vi "SwerveDrivePoseEst_UpdateWithTime.vi"(6 "ModulePositions":T1[](array[typedef]) {"Angle"."SIN" format="%13.4f"; "Angle"."COS" format="%13.4f"; "Angle"."VALUE" format="%13.4f"}, 8 "SweveModuleStates":T3[](array[typedef]) {"Angle"."SIN" format="%13.4f"; "Angle"."COS" format="%13.4f"; "Angle"."VALUE" format="%13.4f"}, 9 "GyroAngle":T2={"VALUE"=0.0, "COS"=1.0, "SIN"=0.0} {"SIN" format="%13.4f"; "COS" format="%13.4f"; "VALUE" format="%13.4f"}, 10 "CurrentTimeSeconds":dbl, 11 "in SwerveDrivePoseEstimate":T6={"M_VisionContR"=[], "m_nominal_dT"=0.0, "m_PrevTime_Sec"=0.0, "m_GyroOffset"={"VALUE"=0.0, "COS"=1.0, "SIN"=0.0}, "m_PrevAngle"={"VALUE"=0.0, "COS"=1.0, "SIN"=0.0}, "m_Observer"={"m_P"=[], "m_xHat"=[], "States"=0, "Outputs"=0, "m_ContR"=[], "m_ContQ"=[], "m_SigmasF"=[], "m_dT_Sec"=0.0, "MERWE_SCALED_SIGMA_PTS"={"m_Wm"=[], "States"=0, "Alpha"=0.0, "m_Wc"=[], "Kappa"=0}, "meanFuncX"=refnum, "meanFuncY"=refnum, "residualFuncX"=refnum, "residualFuncY"=refnum, "addFuncX"=refnum, "addFuncXExtra"=variant, "residualFuncYExtra"=variant, "residualFuncXExtra"=variant, "MeanFuncYExtra"=variant, "MeanFuncXExtra"=variant, "Inputs"=0}, "m_kinematics"={"NumModules"=0, "InverseKinematics"=[], "ForwardKinematics"=[], "Modules"=[], "PrevCoR"={"X"=0.0, "Y"=0.0}, "SavedModuleStates"=[]}, "Pose_Buffer"={"TimeStamps"=[], "Pose"=[], "Min_TimeStamp"=0.0, "Max_TimeStamp"=0.0, "ItemCount"=0, "MaxBufferTime"=0.0}, "States"=0, "Inputs"=0, "Outputs"=0} {"Pose_Buffer"."Pose"."ROTATION"."SIN" format="%13.4f"; "Pose_Buffer"."Pose"."ROTATION"."COS" format="%13.4f"; "Pose_Buffer"."Pose"."ROTATION"."VALUE" format="%13.4f"; "Pose_Buffer"."Pose"."TRANSLATION"."Y" format="%14.3f"; "Pose_Buffer"."Pose"."TRANSLATION"."X" format="%14.3f"; "m_kinematics"."SavedModuleStates"."Angle"."SIN" format="%13.4f"; "m_kinematics"."SavedModuleStates"."Angle"."COS" format="%13.4f"; "m_kinematics"."SavedModuleStates"."Angle"."VALUE" format="%13.4f"; "m_kinematics"."PrevCoR"."Y" format="%14.3f"; "m_kinematics"."PrevCoR"."X" format="%14.3f"; "m_kinematics"."Modules"."Y" format="%14.3f"; "m_kinematics"."Modules"."X" format="%14.3f"; "m_PrevAngle"."SIN" format="%13.4f"; "m_PrevAngle"."COS" format="%13.4f"; "m_PrevAngle"."VALUE" format="%13.4f"; "m_GyroOffset"."SIN" format="%13.4f"; "m_GyroOffset"."COS" format="%13.4f"; "m_GyroOffset"."VALUE" format="%13.4f"}) -> (0 "Error":bool, 2 "Estimated Pose":T4 {"ROTATION"."SIN" format="%13.4f"; "ROTATION"."COS" format="%13.4f"; "ROTATION"."VALUE" format="%13.4f"; "TRANSLATION"."Y" format="%14.3f"; "TRANSLATION"."X" format="%14.3f"}, 3 "Out SwerveDrivePoseEstimate":T6={"M_VisionContR"=[], "m_nominal_dT"=0.0, "m_PrevTime_Sec"=0.0, "m_GyroOffset"={"VALUE"=0.0, "COS"=1.0, "SIN"=0.0}, "m_PrevAngle"={"VALUE"=0.0, "COS"=1.0, "SIN"=0.0}, "m_Observer"={"m_P"=[], "m_xHat"=[], "States"=0, "Outputs"=0, "m_ContR"=[], "m_ContQ"=[], "m_SigmasF"=[], "m_dT_Sec"=0.0, "MERWE_SCALED_SIGMA_PTS"={"m_Wm"=[], "States"=0, "Alpha"=0.0, "m_Wc"=[], "Kappa"=0}, "meanFuncX"=refnum, "meanFuncY"=refnum, "residualFuncX"=refnum, "residualFuncY"=refnum, "addFuncX"=refnum, "addFuncXExtra"=variant, "residualFuncYExtra"=variant, "residualFuncXExtra"=variant, "MeanFuncYExtra"=variant, "MeanFuncXExtra"=variant, "Inputs"=0}, "m_kinematics"={"NumModules"=0, "InverseKinematics"=[], "ForwardKinematics"=[], "Modules"=[], "PrevCoR"={"X"=0.0, "Y"=0.0}, "SavedModuleStates"=[]}, "Pose_Buffer"={"TimeStamps"=[], "Pose"=[], "Min_TimeStamp"=0.0, "Max_TimeStamp"=0.0, "ItemCount"=0, "MaxBufferTime"=0.0}, "States"=0, "Inputs"=0, "Outputs"=0} {"Pose_Buffer"."Pose"."ROTATION"."SIN" format="%13.4f"; "Pose_Buffer"."Pose"."ROTATION"."COS" format="%13.4f"; "Pose_Buffer"."Pose"."ROTATION"."VALUE" format="%13.4f"; "Pose_Buffer"."Pose"."TRANSLATION"."Y" format="%14.3f"; "Pose_Buffer"."Pose"."TRANSLATION"."X" format="%14.3f"; "m_kinematics"."SavedModuleStates"."Angle"."SIN" format="%13.4f"; "m_kinematics"."SavedModuleStates"."Angle"."COS" format="%13.4f"; "m_kinematics"."SavedModuleStates"."Angle"."VALUE" format="%13.4f"; "m_kinematics"."PrevCoR"."Y" format="%14.3f"; "m_kinematics"."PrevCoR"."X" format="%14.3f"; "m_kinematics"."Modules"."Y" format="%14.3f"; "m_kinematics"."Modules"."X" format="%14.3f"; "m_PrevAngle"."SIN" format="%13.4f"; "m_PrevAngle"."COS" format="%13.4f"; "m_PrevAngle"."VALUE" format="%13.4f"; "m_GyroOffset"."SIN" format="%13.4f"; "m_GyroOffset"."COS" format="%13.4f"; "m_GyroOffset"."VALUE" format="%13.4f"})   [LabVIEW 2019, in "Trajectory_Library.lvlib"]
doc: "This set of functions is deprecated. Suggest using the new Swerve Drive Pose Est 2 instead.\n\nUpdates the the Unscented Kalman Filter using only wheel encoder information. This should be called every loop, and the correct loop period must be passed into the constructor of this class.\n \nInputs:\n - SwervePoseEst -- Data cluster containing SwervePoseEst data\n - currentTimeSeconds Time at which this method was called, in seconds.\n - gyroAngle The current gyroscope angle.\n - moduleStates The current velocities and rotations of the swerve modules.\n - modulePositions -- The current distance measurements and rotations of the swerve modules.\n\nOutputs:\n - outSwevePoseEst -- Updated data cluster \n - EstimatedPose -- The estimated pose of the robot in meters.\n - Error -- If TRUE, an error occured."
uses:
  Trajectory_Library.lvlib
  TypeDef/SWERVE_DRIVE_POSE_EST.ctl
  <vilib>/Analysis/Matrix/Datatypes/RealMatrix.ctl
  TypeDef/ROTATION2D.ctl
  TypeDef/UNSCENTED_KALMAN_FILTER.ctl
  TypeDef/MERWE_SCALED_SIGMA_PTS.ctl
  TypeDef/CALLBACK_FUNC_TYPE.ctl
  TypeDef/SWERVE_DRIVE_KINEMATICS.ctl
  TypeDef/TRANSLATION2D.ctl
  TypeDef/SWERVE_DRIVE_MODULE_STATE.ctl
  TypeDef/TIME_INTERPOLATABLE_POSE2D.ctl
  TypeDef/POSE2D.ctl
  TypeDef/SWERVE_DRIVE_MODULE_POSITION.ctl
  Rotation2d_RotateBy.vi
  MatBuilder_Create.vi
  Rotation2d_UnaryMinus.vi
  VI/TimeInterpPose2d_CleanUp.vi
  Rotation2d_CreateXY.vi
  Rotation2d_CreateAngle.vi
  Util_CalcDist.vi
  <vilib>/gmath/interp.llb/Search Ordered Table.vi
  <vilib>/Analysis/Matrix/NI_Matrix.lvlib
panel:
  # "<3, 3>"
  # "State Estimate <Statess,1>"
  # "<States, States>"
  # "<States, ?>"
  # "<Statess,  States>"
  # "<Outputs, Outputs>"
  # "<?, 1>"
  # "<?, 1>"
  # "<3, 3>"
  # "State Estimate <Statess,1>"
  # "<States, States>"
  # "<States, ?>"
  # "<Statess,  States>"
  # "<Outputs, Outputs>"
  # "<?, 1>"
  # "<?, 1>"
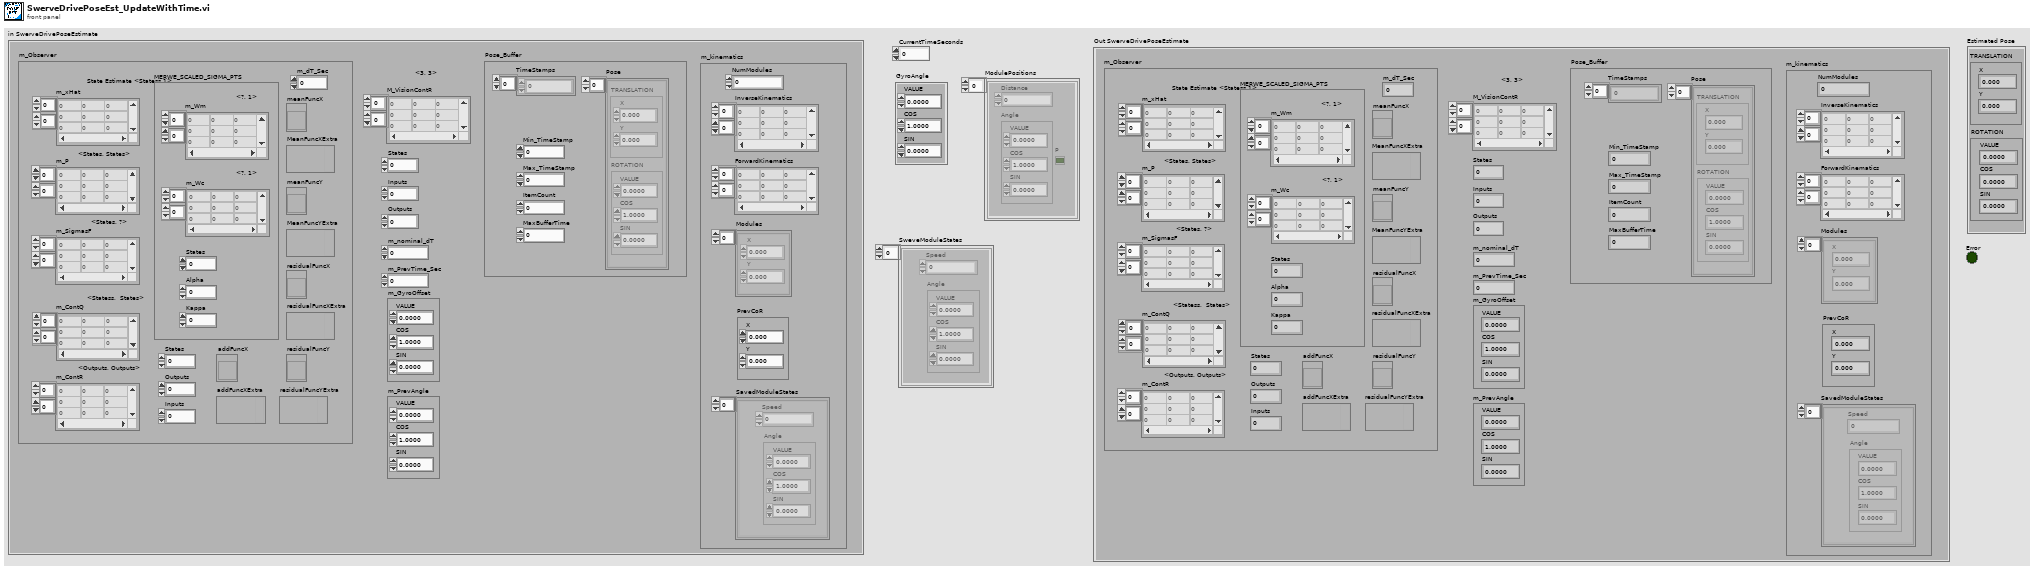
[diagram p1: front panel]
types:
  T1 = typedef "Trajectory_Library.lvlib/SWERVE_DRIVE_MODULE_POSITION.ctl" = cluster{"Distance":dbl, "Angle":T2, "P":bool}
  T2 = typedef "Trajectory_Library.lvlib/ROTATION2D.ctl" = cluster{"VALUE":dbl, "COS":dbl, "SIN":dbl}
  T3 = typedef "Trajectory_Library.lvlib/SWERVE_DRIVE_MODULE_STATE.ctl" = cluster{"Speed":dbl, "Angle":T2}
  T4 = typedef "Trajectory_Library.lvlib/POSE2D.ctl" = cluster{"TRANSLATION":T5, "ROTATION":T2}
  T5 = typedef "Trajectory_Library.lvlib/TRANSLATION2D.ctl" = cluster{"X":dbl, "Y":dbl}
  T6 = typedef "Trajectory_Library.lvlib/SWERVE_DRIVE_POSE_EST.ctl" = cluster{"M_VisionContR":T7, "m_nominal_dT":dbl, "m_PrevTime_Sec":dbl, "m_GyroOffset":T2, "m_PrevAngle":T2, "m_Observer":T8, "m_kinematics":T11, "Pose_Buffer":T12, "States":i32, "Inputs":i32, "Outputs":i32}
  T7 = typedef "NI_Matrix.lvlib/RealMatrix.ctl" = dbl[][]
  T8 = typedef "Trajectory_Library.lvlib/UNSCENTED_KALMAN_FILTER.ctl" = cluster{"m_P":T7, "m_xHat":T7, "States":i32, "Outputs":i32, "m_ContR":T7, "m_ContQ":T7, "m_SigmasF":T7, "m_dT_Sec":dbl, "MERWE_SCALED_SIGMA_PTS":T9, "meanFuncX":T10, "meanFuncY":T10, "residualFuncX":T10, "residualFuncY":T10, "addFuncX":T10, "addFuncXExtra":variant, "residualFuncYExtra":variant, "residualFuncXExtra":variant, "MeanFuncYExtra":variant, "MeanFuncXExtra":variant, "Inputs":i32}
  T9 = typedef "Trajectory_Library.lvlib/MERWE_SCALED_SIGMA_PTS.ctl" = cluster{"m_Wm":T7, "States":i32, "Alpha":dbl, "m_Wc":T7, "Kappa":i32}
  T10 = typedef "Trajectory_Library.lvlib/CALLBACK_FUNC_TYPE.ctl" = refnum<vi>
  T11 = typedef "Trajectory_Library.lvlib/SWERVE_DRIVE_KINEMATICS.ctl" = cluster{"NumModules":i32, "InverseKinematics":T7, "ForwardKinematics":T7, "Modules":T5[], "PrevCoR":T5, "SavedModuleStates":T3[]}
  T12 = typedef "Trajectory_Library.lvlib/TIME_INTERPOLATABLE_POSE2D.ctl" = cluster{"TimeStamps":dbl[], "Pose":T4[], "Min_TimeStamp":dbl, "Max_TimeStamp":dbl, "ItemCount":i32, "MaxBufferTime":dbl}
  T13 = typedef "Trajectory_Library.lvlib/CHASSIS_SPEEDS.ctl" = cluster{"vX":dbl, "vY":dbl, "vOmega":dbl}
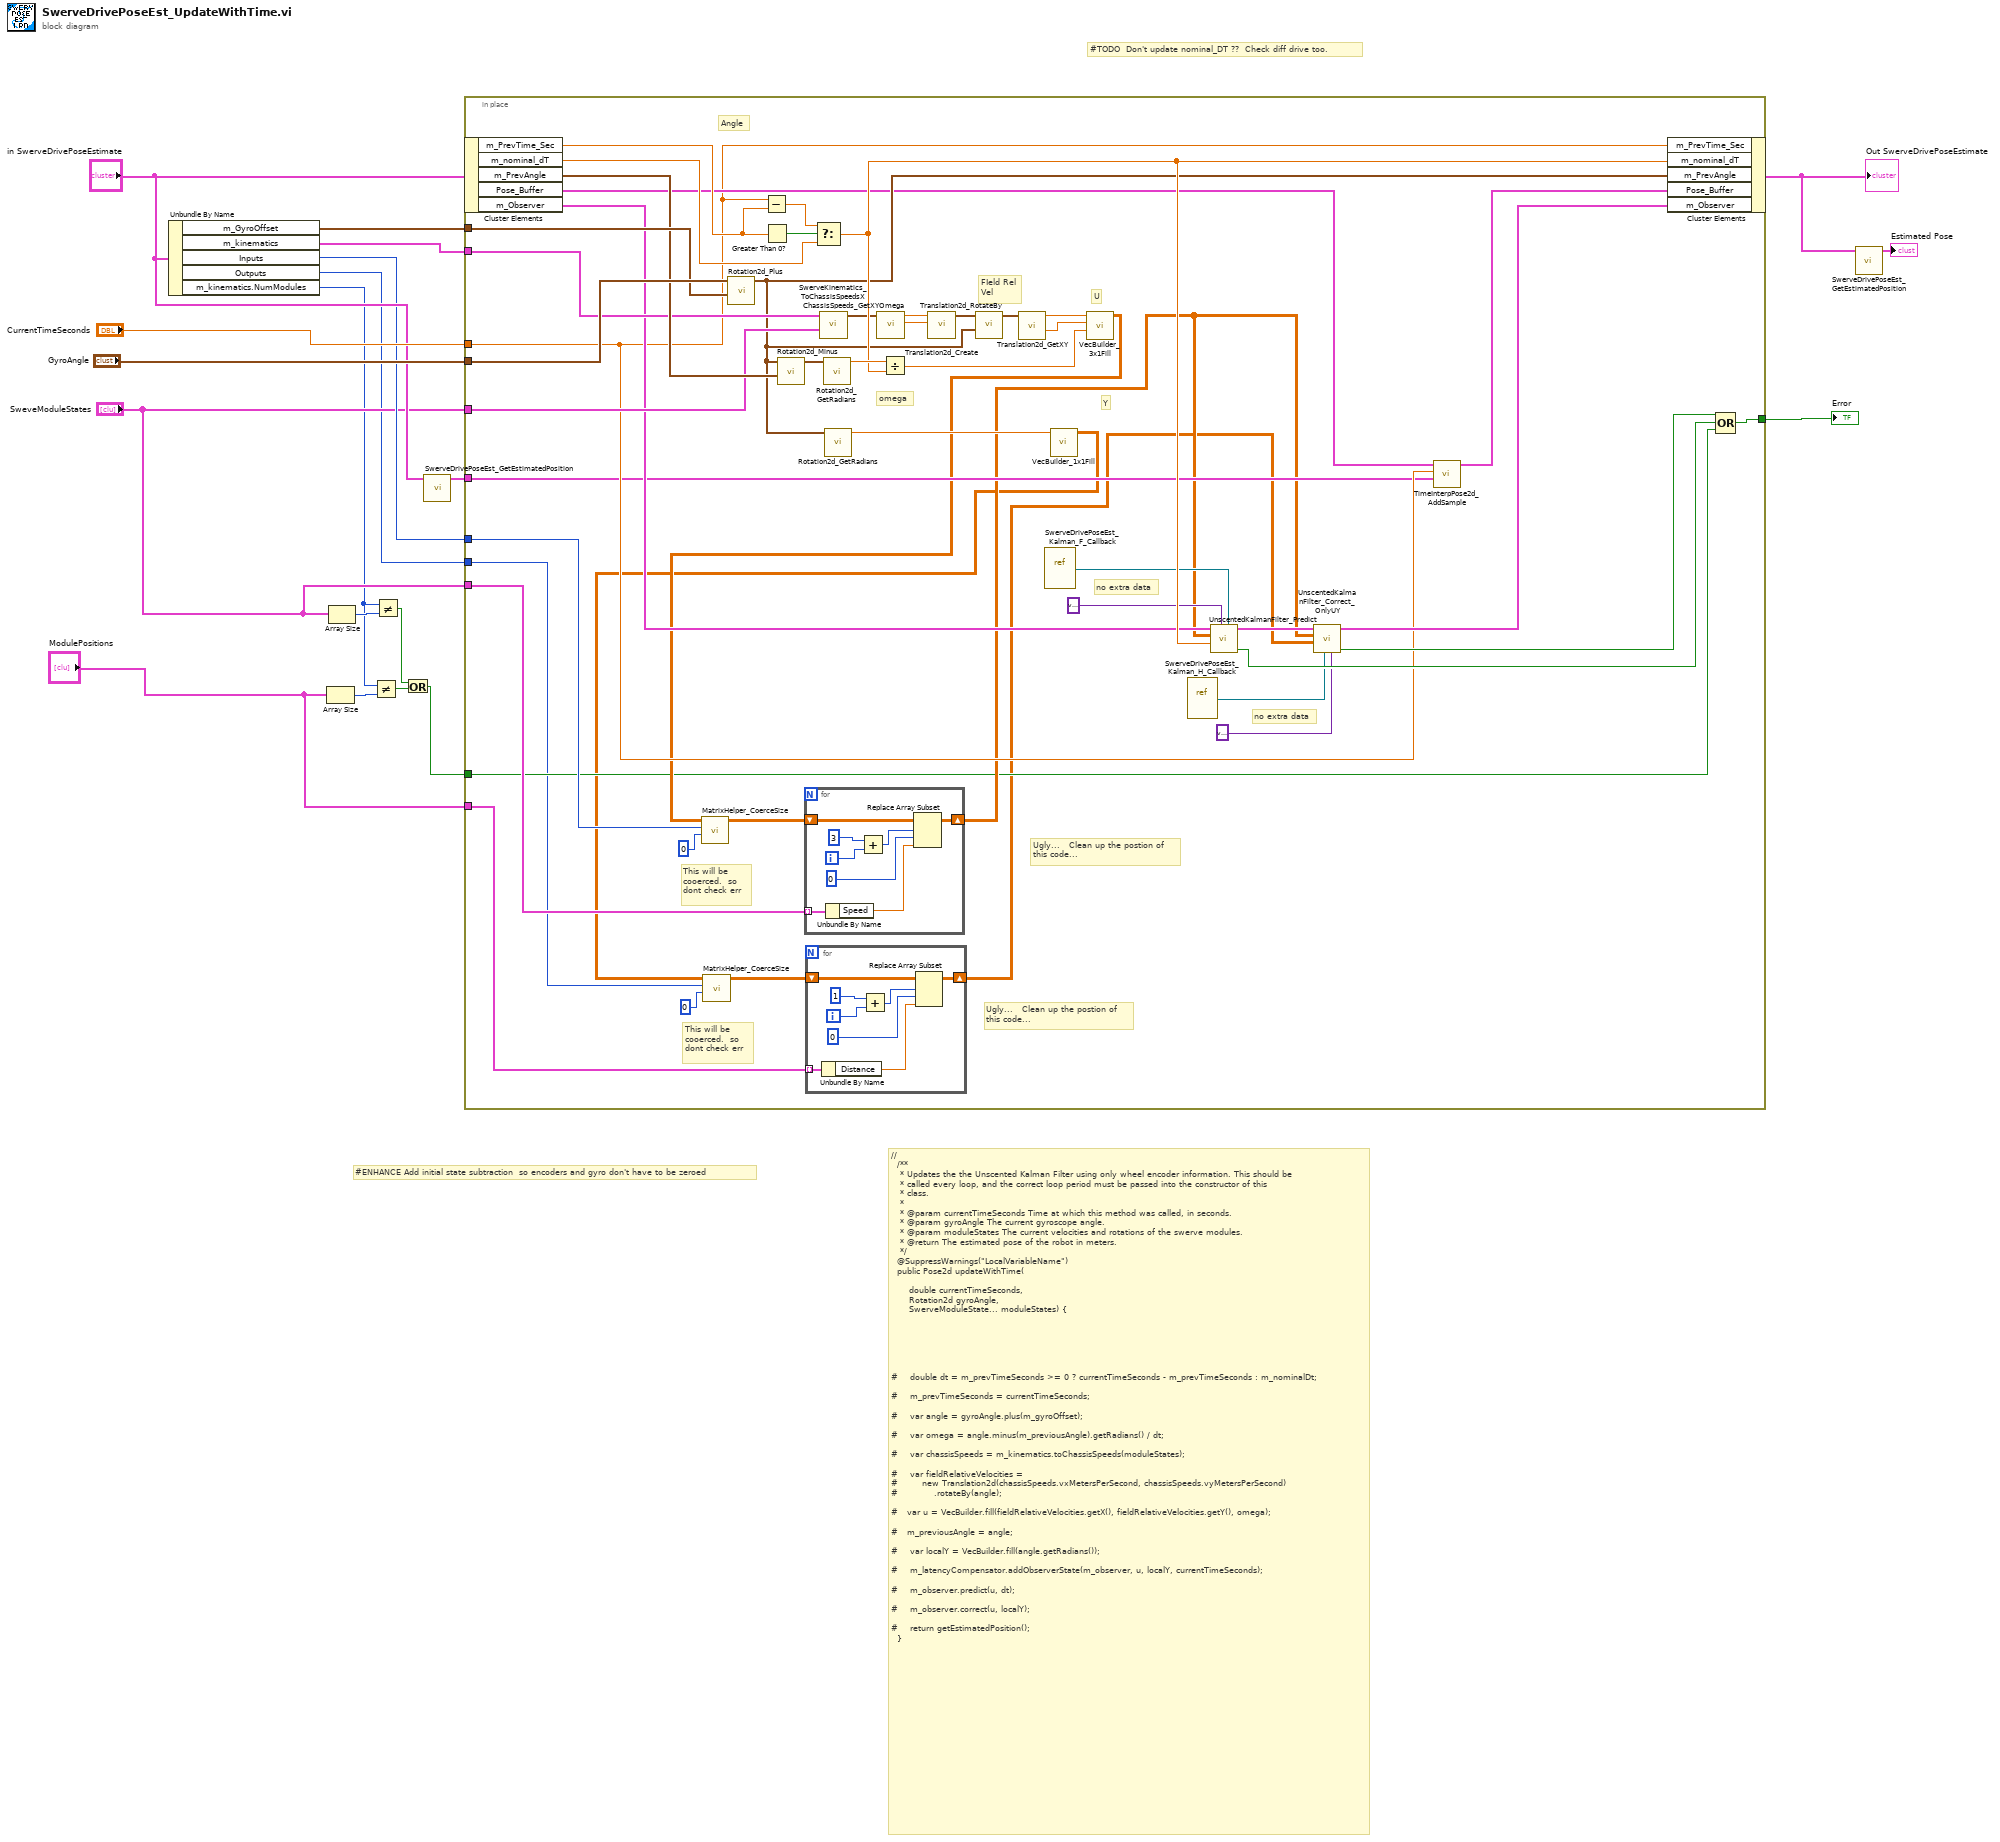
[diagram p0: block diagram]
diagram:
  # "#TODO  Don't update nominal_DT ??  Check diff drive too."
  # "#ENHANCE Add initial state subtraction  so encoders and gyro don't have to be zeroed"
  # "//\n  /**\n   * Updates the the Unscented Kalman Filter using only wheel encoder information. This should be\n   * called every loop, and the correct loop period must be passed into the constructor of this\n   * class.\n   *\n   * @param currentTimeSeconds Time at which this method was called, in seconds.\n   * @param gyroAngle The current gyroscope angle.\n   * @param moduleStates The current velocities and rotations of the swerve modules.\n   * @return The estimated pose of the robot in meters.\n   */\n  @SuppressWarnings(\"LocalVariableName\")\n  public Pose2d updateWithTime(\n\n      double currentTimeSeconds, \n      Rotation2d gyroAngle, \n      SwerveModuleState... moduleStates) {\n\n\n\n\n\n\n#    double dt = m_prevTimeSeconds >= 0 ? currentTimeSeconds - m_prevTimeSeconds : m_nominalDt;\n\n#    m_prevTimeSeconds = currentTimeSeconds;\n\n#    var angle = gyroAngle.plus(m_gyroOffset);\n\n#    var omega = angle.minus(m_previousAngle).getRadians() / dt;\n\n#    var chassisSpeeds = m_kinematics.toChassisSpeeds(moduleStates);\n\n#    var fieldRelativeVelocities =\n#        new Translation2d(chassisSpeeds.vxMetersPerSecond, chassisSpeeds.vyMetersPerSecond)\n#            .rotateBy(angle);\n\n#   var u = VecBuilder.fill(fieldRelativeVelocities.getX(), fieldRelativeVelocities.getY(), omega);\n \n#   m_previousAngle = angle;\n\n#    var localY = VecBuilder.fill(angle.getRadians());\n\n#    m_latencyCompensator.addObserverState(m_observer, u, localY, currentTimeSeconds);\n\n#    m_observer.predict(u, dt);\n\n#    m_observer.correct(u, localY);\n\n#    return getEstimatedPosition();\n  }"
  n1 = Unbundle By Name("in SwerveDrivePoseEstimate") -> ("m_GyroOffset"=w17:T2, "m_kinematics"=w13:T11, "Inputs"=w10:i32, "Outputs"=w2:i32, "m_kinematics.NumModules"=w3:i32)
  n2 = Array Size(array="ModulePositions") -> (size(s)=w9:i32)
  n3 = Array Size(array="SweveModuleStates") -> (size(s)=w8:i32)
  n4 = Not Equal?(x=w3, y=w9) -> (x != y?=w7:bool)
  n5 = Not Equal?(x=w3, y=w8) -> (x != y?=w6:bool)
  n6 = Or(x=w6, y=w7) -> (x .or. y?=w5:bool)
  n7 = call "SwerveDrivePoseEst_GetEstimatedPosition.vi"("in SwerveDrivePoseEstimate"="in SwerveDrivePoseEstimate") -> ("Estimated Pose"=w11:T4)  [unwired: 10 in]
  n8 = in-place {
    in-place-border: "CurrentTimeSeconds" -> [w35]
    in-place-border: "GyroAngle" -> [w65]
    in-place-border: w17 -> [w64]
    in-place-border: [w57] -> w14
    in-place-border: w13 -> [w51]
    in-place-border: "SweveModuleStates" -> [w50]
    in-place-border: w11 -> [w34]
    in-place-border: w10 -> [w30]
    in-place-border: "SweveModuleStates" -> [w29]
    in-place-border: w5 -> [w26]
    in-place-border: w2 -> [w23]
    in-place-border: "ModulePositions" -> [w22]
    # "Ugly...   Clean up the postion of\nthis code..."
    # "This will be\ncooerced.  so\ndont check err"
    # "Ugly...   Clean up the postion of\nthis code..."
    # "This will be\ncooerced.  so\ndont check err"
    # "FIeld Rel\nVel"
    # "omega"
    # "Angle"
    # "no extra data"
    # "no extra data"
    # "Y"
    # "U"
    n9 = in-place-cluster #1("in SwerveDrivePoseEstimate") -> ("m_PrevTime_Sec"=w67:dbl, "m_nominal_dT"=w62:dbl, "m_PrevAngle"=w52:T2, "Pose_Buffer"=w37:T12, "m_Observer"=w38:T8)
    n10 = call "Rotation2d_Plus.vi"("other ROTATION"=w64, "in ROTATION"=w65) -> ("out ROTATION"=w46:T2)  [unwired: 9 in]
    n11 = Subtract(x=w35, y=w67) -> (x-y=w66:dbl)
    n12 = Greater Than 0?(x=w67) -> (x > 0?=w68:bool)
    n13 = call "Rotation2d_Minus.vi"("other ROTATION"=w52, "in ROTATION"=w46) -> ("out ROTATION"=w63:T2)  [unwired: 9 in]
    n14 = Select(t=w66, s=w68, f=w62) -> (s? t:f=w56:dbl)
    n15 = call "SwerveKinematics_ToChassisSpeedsX.vi"("WheelStates"=w50, "in SWERVE_DRIVE_KINEMATICS"=w51) -> ("Chassis Speed"=w33:T13)  [unwired: 9 in]
    n16 = call "Rotation2d_GetRadians.vi"("in ROTATION"=w63) -> ("AngleRadians"=w61:dbl)  [unwired: 10 in]
    n17 = call "Rotation2d_GetRadians.vi"("in ROTATION"=w46) -> ("AngleRadians"=w41:dbl)  [unwired: 10 in]
    n18 = call "ChassisSpeeds_GetXYOmega.vi"("CHASSIS"=w33) -> ("vY"=w48:dbl, "vX"=w49:dbl)  [unwired: 8 in, 1 out]
    n19 = Divide(x=w61, y=w56) -> (x/y=w42:dbl)
    n20 = call "Translation2d_Create.vi"("Y"=w48, "X"=w49) -> ("TRANSLATION"=w47:T5)  [unwired: 9 in]
    n21 = call "Translation2d_RotateBy.vi"("other Rotation"=w46, "In Translation"=w47) -> ("Out Translation"=w45:T5)  [unwired: 9 in]
    n22 = call "Translation2d_GetXY.vi"("In Translation"=w45) -> ("Y"=w43:dbl, "X"=w44:dbl)  [unwired: 9 in]
    n23 = vi-ref "SwerveDrivePoseEst_Kalman_F_Callback.vi"() -> (w40:refnum<vi>)
    n24 = call "VecBuilder_1x1Fill.vi"("R0_C0"=w41) -> ("output matrix"=w21:T7)  [unwired: 10 in]
    n25 = call "MatrixHelper_CoerceSize.vi"("Columns"=0, "Rows"=w23, "input matrix"=w21) -> ("output matrix"=w25:T7)  [unwired: 7 in, 1 out]
    n26 = for {
      tunnel: w22 -> [w76] mode=indexing
      shift-right: [w69] -> w20
      shift-left: w25 -> [w73]
      i -> [w74]
      n27 = Unbundle By Name(w76) -> ("Distance"=w70:dbl)
      n28 = Add(x=1 ("States"), y=w74) -> (x+y=w72:i32)
      n29 = Replace Array Subset(array=w73, new element=w70, index (row)=w72, index (col)=0 ("disabled index (col)")) -> (w69:T7)
    }
    n30 = call "VecBuilder_3x1Fill.vi"("R2"=w42, "R1"=w43, "R0"=w44) -> ("output matrix"=w28:T7)  [unwired: 8 in]
    n31 = call "MatrixHelper_CoerceSize.vi"("Columns"=0, "Rows"=w30, "input matrix"=w28) -> ("output matrix"=w32:T7)  [unwired: 7 in, 1 out]
    n32 = for {
      tunnel: w29 -> [w84] mode=indexing
      shift-right: [w77] -> w27
      shift-left: w32 -> [w81]
      i -> [w82]
      n33 = Unbundle By Name(w84) -> ("Speed"=w78:dbl)
      n34 = Add(x=3 ("States"), y=w82) -> (x+y=w80:i32)
      n35 = Replace Array Subset(array=w81, new element=w78, index (row)=w80, index (col)=0 ("disabled index (col)")) -> (w77:T7)
    }
    n36 = vi-ref "SwerveDrivePoseEst_Kalman_H_Callback.vi"() -> (w39:refnum<vi>)
    n37 = call "UnscentedKalmanFilter_Predict.vi"("f_Func"=w40, "F_Func_ExtraData"=variant, "dT_Seconds"=w56, "U"=w27, "in UnscentedKalmanFiilter"=w38) -> ("Error"=w58:bool, "out UnscentedKalmanFiilter"=w60:T8)  [unwired: 5 in]
    n38 = call "UnscentedKalmanFilter_Correct_OnlyUY.vi"("H_ExtraData"=variant ("F_Func_ExtraData"), "H_Func"=w39, "Y"=w20, "U"=w27, "in UnscentedKalmanFiilter"=w60) -> ("Error"=w59:bool, "out UnscentedKalmanFiilter"=w53:T8)  [unwired: 5 in]
    n39 = call "TimeInterpPose2d_AddSample.vi"("Pose"=w34, "TimeStamp"=w35, "in TimeInterpPose"=w37) -> ("out TimeInterpPose"=w36:T12)  [unwired: 7 in, 1 out]
    n40 = in-place-cluster #1("m_PrevTime_Sec"=w35, "m_nominal_dT"=w56, "m_PrevAngle"=w46, "Pose_Buffer"=w36, "m_Observer"=w53) -> (w16:T6)
    n41 = Compound Arithmetic op=OR(w59, w58, w26) -> (w57:bool)
  }
  "Out SwerveDrivePoseEstimate" <- w16
  "Error" <- w14
  n42 = call "SwerveDrivePoseEst_GetEstimatedPosition.vi"("in SwerveDrivePoseEstimate"=w16) -> ("Estimated Pose"=→"Estimated Pose":T4)  [unwired: 10 in]
